vi "ex_PluginTemplateConfig.vi"(11 "Parameters in":string) -> (3 "Parameters out":string)   [LabVIEW 2020]
panel:
  in  "error in (no error)":errorcluster
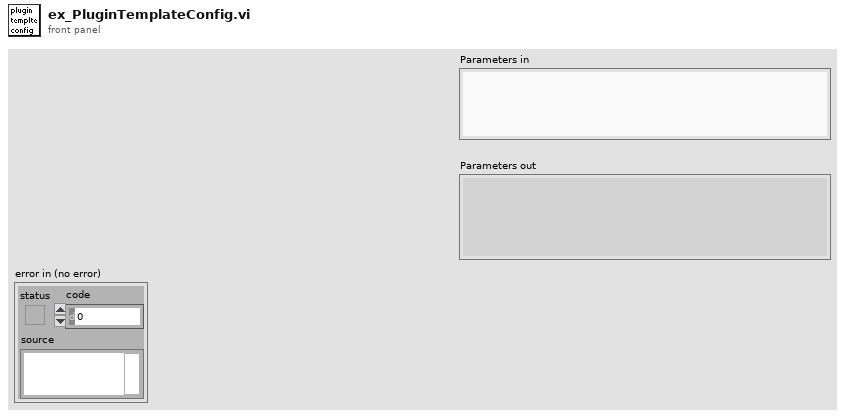
[diagram p1: front panel]
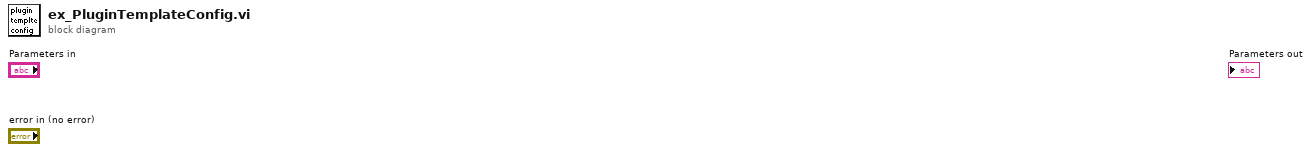
[diagram p0: block diagram]
diagram:
